vi "Image DAQ.vi"() -> ()   [LabVIEW 2020]
uses:
  SubVIs/MASTER.ctl
  SubVIs/Constants.ctl
  SubVIs/QBundle.ctl
  SubVIs/Queue.ctl
  SubVIs/Image data.ctl
  <vilib>/userdefined/High Color/IMAQdx.ctl
  <vilib>/vision/Image Controls.llb/IMAQ Image.ctl
  SubVIs/Image QBundle.ctl
panel:
  in  "Crosshairs":bool
  in  "Color Palette":u16(ring) items=["Grayscale U8", "False Color", "Overexposed"]
  in  "Exposure time [us]":dbl format="%#_10g"
  out "C2 Image out":T1(plugin-control) caption="Image Out"
  out "C2 Model Name":string
  in  "Camera 2":refnum<k21> caption="IMAQdx Session"
  out "C1 Image out":T1(plugin-control) caption="Image Out"
  out "C1 Model Name":string
  in  "Camera 1":refnum<k21> caption="IMAQdx Session"
  out "Image count":dbl
  in  "Digital output task":refnum<k21>
  in  "File type":string(combo)
  in  "Analog input task":refnum<k21>
  in  "Chart display tabs":T2(tab) caption="Display tabs"
  out "Analog Signals - Raw voltage":cluster{"Raw data[0]":dbl, "Raw data[1]":dbl}(graph)
  out "Analog Signals - Engineering units":cluster{"Engr data[0]":dbl, "Engr data[1]":dbl}(graph)
  in  "Scale (0) & Offset (1)":dbl[][](array[numeric])
  in  "AS #":string[](array[string])
  out "Channel Name":string[](array[string])
  out "Zero [V]":dbl[](array[numeric])
  out "Scale (0) & Offset (1)":dbl[][](array[numeric])
  in  "Enable":bool
  in  "Zero button":bool
  in  "Zero Signal [V]":dbl[](array[numeric])
  out "Analog Signals - Zero voltage":cluster{"Raw data[0]":dbl, "Raw data[1]":dbl}(graph)
  in  "Time":u16(ring) items=["Absolute time", "Relative time"]
  out "Timestamp [s]":dbl
  in  "Record data":bool
  in  "Sampling frequency [Hz]":dbl format="%#_10g"
  in  "Stop":bool
  in  "File Folder":path
  # "Records analog data and triggers cameras at specified rate. Writes raw voltage data to CSV file. Exports images as PNG files."
  # "Recording parameters- do not change while program is running"
  # "Recording indicators"
  # "Recording controls"
  # "Camera controls"
  # "Instructions: \n1. Click file icon to select file folder\n2. Select file type. Default is a CSV file. \n3. Set the sample frequency for data acquisition. Default is 1 Hz. \n4. Select analog input task\n5. Select digital output task\n6. Select type of timestamp\n7. Run program with white arrow in tool bar\n8. Use controls to record data adn trigger cameras\n9. Zero raw data on 'ZERO' tab. Zeroed data is recorded as raw data when 'Enable' button is on. \n10. Scale chart to engineering units on 'ENGR' tab\n11. Record AS number of equipment on 'Channel Info' tab\n12. Stop program with 'STOP' button"
  # "Note: If editing number of channels in DAQmx task, seek help from Instrumentation team. Chart cluster size & historical data constant must be adjusted in back panel."
  # "Scale [Unit/V] & Offset [Unit]"
  # "Channel Information"
  # "Offset [Unit]"
  # "Scale [Unit/V]"
  # "Zeroed data is recorded as raw data when Enable button is on."
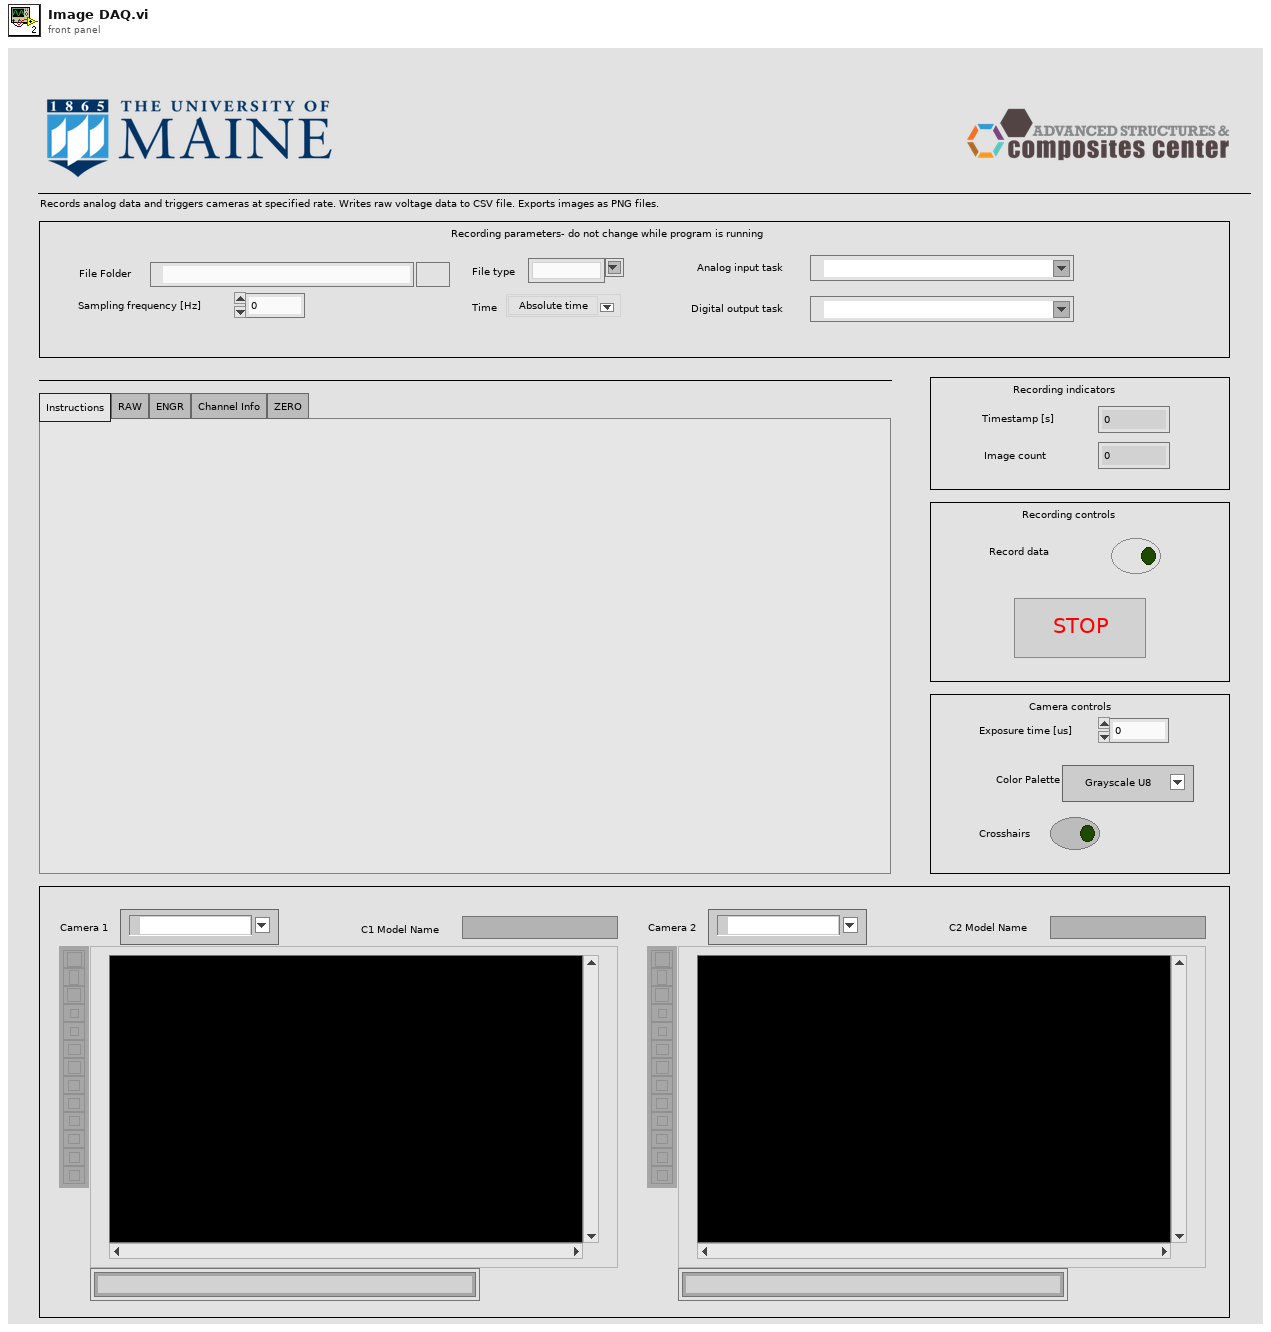
[diagram p1: front panel]
types:
  T1 = typedef "IMAQ Image.ctl" = refnum<image>
  T2 = enum32{"Instructions", "RAW", "ENGR", "Channel Info", "ZERO"}
  T3 = typedef "MASTER.ctl" = cluster{"Constants":T4, "Queue Bundle":T5, "Queue":T6, "Image data":T7, "Image QBundle ":T9}
  T4 = typedef "Constants.ctl" = cluster{"Time":u16, "Samp. freq. [Hz]":dbl, "Samp. per chan.":i32, "Avg. div.":i32, "File path":path, "AI":refnum<k21>, "Loop 1 [Hz]":dbl, "Loop 2 [Hz]":dbl, "Loop 3 [Hz]":dbl, "Loop 1 [ms]":dbl, "Loop 2 [ms]":dbl, "Loop 3 [ms]":dbl, "Q1 buffer size":i32, "Q2 buffer size":i32, "File type":string, "Loop 4 [Hz]":dbl, "Loop 4 [ms]":dbl, "Channel Name":string[], "AS #":string[], "DO":refnum<k21>}
  T5 = typedef "QBundle.ctl" = cluster{"queue 1":refnum<queue>, "error 1":errorcluster, "queue 2":refnum<queue>, "error 2":errorcluster}
  T6 = typedef "Queue.ctl" = cluster{"Enable zero":bool, "Engr data [Unit]":dbl[], "Zero button":bool, "Zero [V]":dbl[], "Timestamp [s]":dbl, "Write sample":bool, "Record control":bool, "Stop":bool, "error":errorcluster, "Raw data [V]\n(all samples)":dbl[][], "Raw data [V]":dbl[], "Loop count":i64, "Initial time [s]":dbl, "Scale (0) & Offset (1)":dbl[][], "Image count":dbl}
  T7 = typedef "Image data.ctl" = cluster{"Camera 1":T8, "Camera 2":T8, "C1 Image out ":T1, "C2 Image out":T1, "C1 Model Name":string, "C2 Model Name":string, "Exposure time [us]":dbl, "Color Palette":u16, "C1 Buffer array":T1[], "Ready":bool, "C2 Buffer array":T1[], "Crosshairs":bool, "Stop":bool}
  T8 = typedef "IMAQdx.ctl" = refnum<k21>
  T9 = typedef "Image QBundle.ctl" = cluster{"queue 1":refnum<queue>, "error 1":errorcluster, "queue 2":refnum<queue>, "error 2":errorcluster}
  T10 = cluster{"Engr data[0]":dbl, "Engr data[1]":dbl}[]
  T11 = cluster{"Engr data [Unit][0]":dbl, "Engr data [Unit][1]":dbl}
  T12 = cluster{"Raw data [V][0]":dbl, "Raw data [V][1]":dbl}
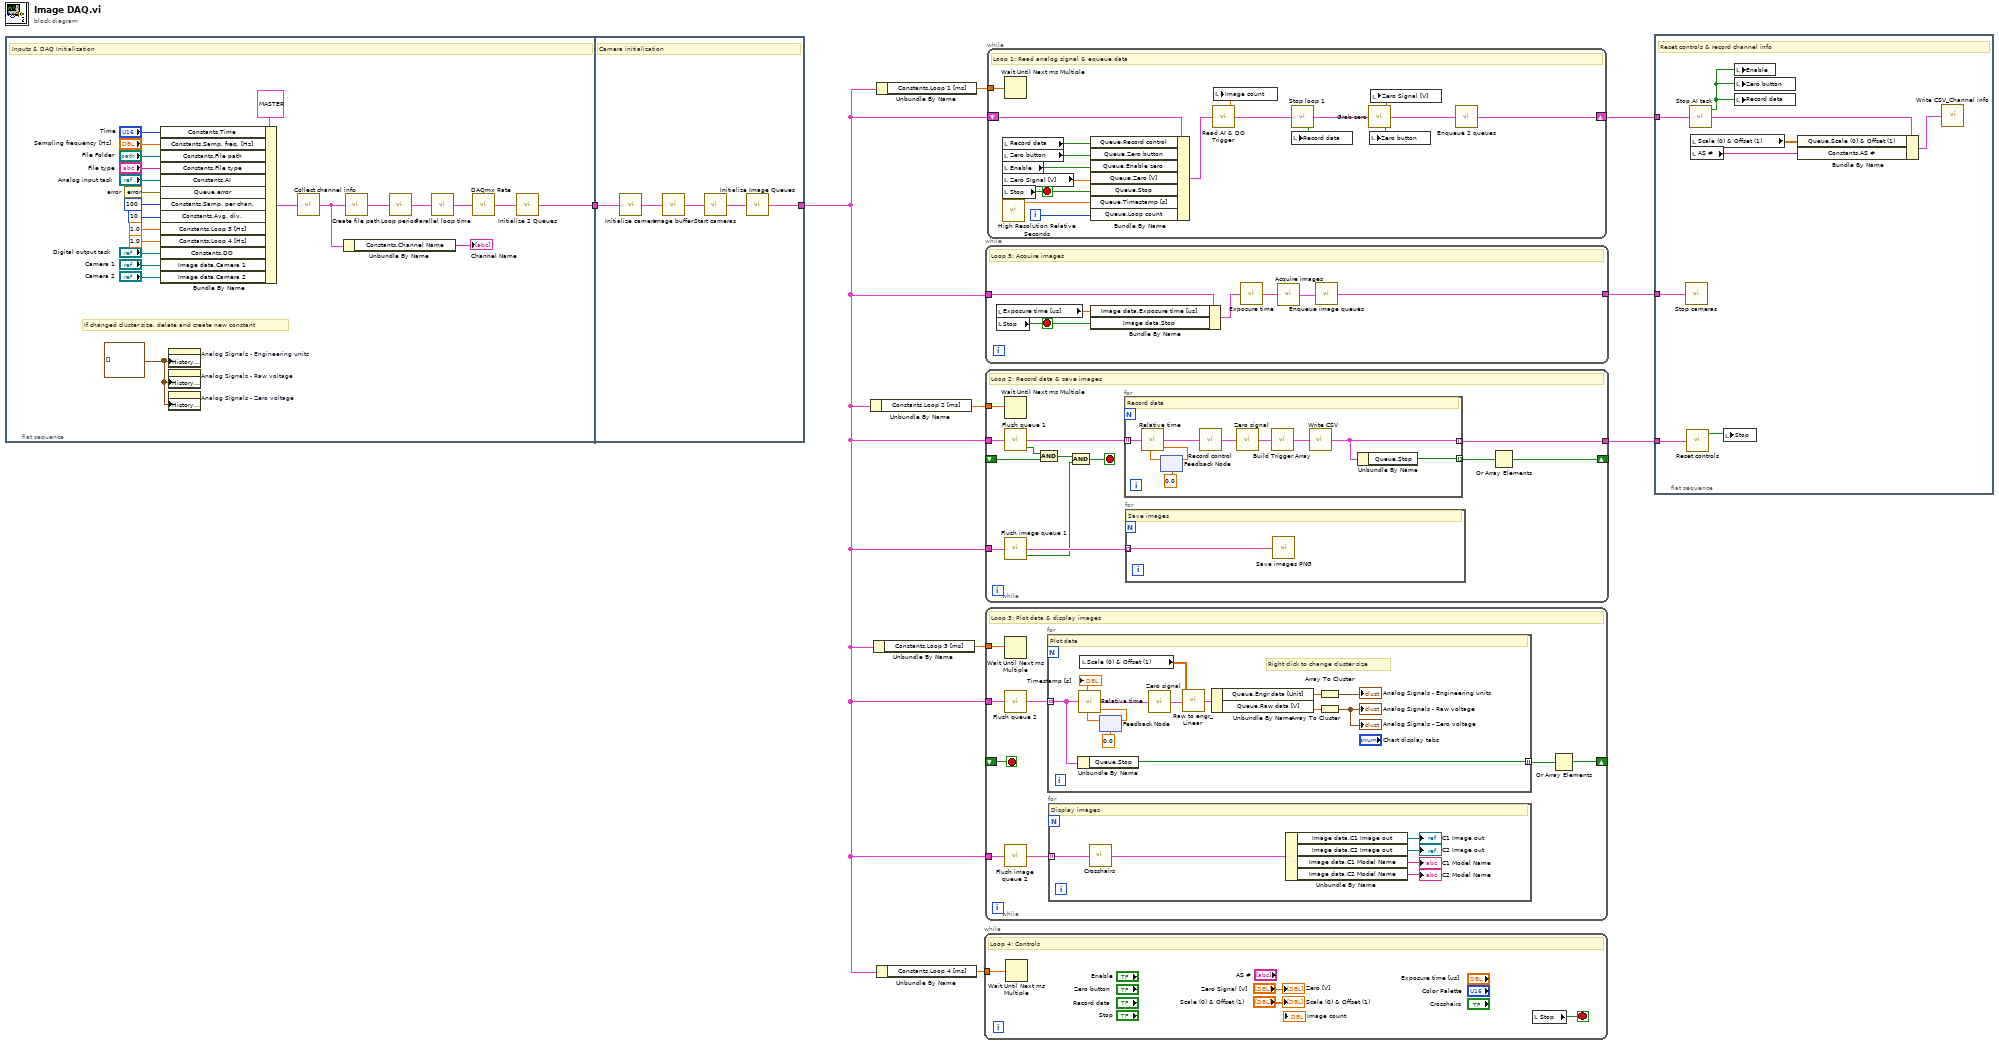
[diagram p0: block diagram]
diagram:
  n1 = flat-sequence {
    tunnel: [w32] -> w3
    tunnel: [w37] -> w1
    tunnel: w3 -> [w36]
    frame #0 {
      w20 = errorcluster {"status"=FALSE, "code"=0, "source"=""}  # error
      w31 = T10 [] ("History Data")
      # "If changed cluster size, delete and create new constant"
      # "Inputs & DAQ Initialization"
      n2 = Bundle By Name(cluster=T3 {"Constants"={"Time"=0, "Samp. freq. [Hz]"=0.0, "Samp. per chan."=0, "Avg. div."=0, "File path"=path "", "AI"="", "Loop 1 [Hz]"=0.0, "Loop 2 [Hz]"=0.0, "Loop 3 [Hz]"=0.0, "Loop 1 [ms]"=0.0, "Loop 2 [ms]"=0.0, "Loop 3 [ms]"=0.0, "Q1 buffer size"=0, "Q2 buffer size"=0, "File type"="", "Loop 4 [Hz]"=0.0, "Loop 4 [ms]"=0.0, "Channel Name"=[], "AS #"=[], "DO"=""}, "Queue Bundle"={"queue 1"=refnum, "error 1"={"status"=FALSE, "code"=0, "source"=""}, "queue 2"=refnum, "error 2"={"status"=FALSE, "code"=0, "source"=""}}, "Queue"={"Enable zero"=FALSE, "Engr data [Unit]"=[], "Zero button"=FALSE, "Zero [V]"=[], "Timestamp [s]"=0.0, "Write sample"=FALSE, "Record control"=FALSE, "Stop"=FALSE, "error"={"status"=FALSE, "code"=0, "source"=""}, "Raw data [V]\n(all samples)"=[], "Raw data [V]"=[], "Loop count"=0, "Initial time [s]"=0.0, "Scale (0) & Offset (1)"=[], "Image count"=0.0}, "Image data"={"Camera 1"="", "Camera 2"="", "C1 Image out "=refnum, "C2 Image out"=refnum, "C1 Model Name"="", "C2 Model Name"="", "Exposure time [us]"=0.0, "Color Palette"=0, "C1 Buffer array"=[], "Ready"=FALSE, "C2 Buffer array"=[], "Crosshairs"=FALSE, "Stop"=FALSE}, "Image QBundle "={"queue 1"=refnum, "error 1"={"status"=FALSE, "code"=0, "source"=""}, "queue 2"=refnum, "error 2"={"status"=FALSE, "code"=0, "source"=""}}} ("Variables"), "Constants.Time"="Time", "Constants.Samp. freq. [Hz]"="Sampling frequency [Hz]", "Constants.File path"="File Folder", "Constants.File type"="File type", "Constants.AI"="Analog input task", "Queue.error"=w20, "Constants.Samp. per chan."=100 ("Samp. per chan."), "Constants.Avg. div."=10 ("Avg. div."), "Constants.Loop 3 [Hz]"=1.0 ("Loop 1 [ms]"), "Constants.Loop 4 [Hz]"=1.0 ("Loop 4 [Hz]"), "Constants.DO"="Digital output task", "Image data.Camera 1"="Camera 1", "Image data.Camera 2"="Camera 2") -> (w15:T3)
      n3 = property on="Analog Signals - Engineering units" class="WFChart (strict)"("History Data"=w31) -> ()  [unwired: 2 in, 2 out]
      n4 = property on="Analog Signals - Raw voltage" class="WFChart (strict)"("History Data"=w31) -> ()  [unwired: 2 in, 2 out]
      n5 = property on="Analog Signals - Zero voltage" class="WFChart (strict)"("History Data"=w31) -> ()  [unwired: 2 in, 2 out]
      n6 = call "Collect channel info.vi"("MASTER in"=w15) -> ("MASTER out"=w13:T3)  [unwired: 4 in]
      n7 = Unbundle By Name(w13) -> ("Constants.Channel Name"=→"Channel Name":string[])
      n8 = call "Create file path.vi"("MASTER in"=w13) -> ("MASTER out"=w29:T3)  [unwired: 4 in]
      n9 = call "Loop period.vi"("MASTER in"=w29) -> ("MASTER out"=w26:T3)  [unwired: 4 in]
      n10 = call "Parallel loop time.vi"("MASTER in"=w26) -> ("MASTER out"=w30:T3)  [unwired: 4 in]
      n11 = call "DAQmx Rate.vi"("MASTER in"=w30) -> ("MASTER out"=w14:T3)  [unwired: 4 in]
      n12 = call "Initialize 2 Queues.vi"("MASTER in"=w14) -> ("MASTER out"=w32:T3)  [unwired: 4 in]
    }
    frame #1 {
      # "Camera initialization"
      n13 = call "Initialize camera.vi"("MASTER in"=w36) -> ("MASTER out"=w35:T3)  [unwired: 4 in]
      n14 = call "Image buffer.vi"("MASTER in"=w35) -> ("MASTER out"=w34:T3)  [unwired: 4 in]
      n15 = call "Start cameras.vi"("MASTER in"=w34) -> ("MASTER out"=w33:T3)  [unwired: 4 in]
      n16 = call "Initialize Image Queues.vi"("MASTER in"=w33) -> ("MASTER out"=w37:T3)  [unwired: 4 in]
    }
  }
  n17 = Unbundle By Name(w1) -> ("Constants.Loop 2 [ms]"=w6:dbl)
  n18 = Unbundle By Name(w1) -> ("Constants.Loop 3 [ms]"=w5:dbl)
  n19 = Unbundle By Name(w1) -> ("Constants.Loop 1 [ms]"=w7:dbl)
  n20 = Unbundle By Name(w1) -> ("Constants.Loop 4 [ms]"=w4:dbl)
  n21 = while {
    tunnel: w4 -> [w41]
    stop <- w38 stop-if-true
    # "Loop 4: Controls"
    n22 = Wait Until Next ms Multiple(millisecond multiple=w41) -> ()  [unwired: 1 out]
    n23 = local read "Stop"() -> (w38:bool)
    "Scale (0) & Offset (1)" <- "Scale (0) & Offset (1)"
    "Zero [V]" <- "Zero Signal [V]"
  }
  n24 = while {
    tunnel: w1 -> [w48]
    tunnel: [w42] -> w2
    stop <- w45 stop-if-true
    # "Loop 5: Acquire images"
    n25 = local read "Exposure time [us]"() -> (w46:dbl)
    n26 = local read "Stop"() -> (w45:bool)
    n27 = Bundle By Name(cluster=w48, "Image data.Exposure time [us]"=w46, "Image data.Stop"=w45) -> (w47:T3)
    n28 = call "Exposure time.vi"("MASTER in"=w47) -> ("MASTER out"=w44:T3)  [unwired: 4 in]
    n29 = call "Acquire images.vi"("MASTER in"=w44) -> ("MASTER out"=w43:T3)  [unwired: 4 in]
    n30 = call "Enqueue image queues.vi"("MASTER in"=w43) -> ("MASTER out"=w42:T3)  [unwired: 4 in]
  }
  n31 = while {
    tunnel: w6 -> [w61]
    shift-right: [w59] -> _
    shift-left: _ -> [w58]
    tunnel: w1 -> [w57]
    tunnel: [w54] -> w8
    tunnel: w1 -> [w52]
    stop <- w51 stop-if-true
    # "Loop 2: Record data & save images"
    n32 = Wait Until Next ms Multiple(millisecond multiple=w61) -> ()  [unwired: 1 out]
    n33 = call "Flush queue 1.vi"("MASTER in"=w57) -> ("MASTER array"=w55:T3[], "Zero elements in queue"=w56:bool)  [unwired: 5 in]
    n34 = call "Flush image queue 1.vi"("MASTER in"=w52) -> ("Zero elements in queue"=w49:bool, "MASTER array"=w53:T3[])  [unwired: 3 in]
    n35 = And(x=w56, y=w58) -> (x .and. y?=w50:bool)
    n36 = And(x=w50, y=w49) -> (x .and. y?=w51:bool)
    n37 = for {
      tunnel: [w72] -> w60 mode=indexing
      tunnel: w55 -> [w69] mode=indexing
      tunnel: [w70] -> w54 mode=indexing
      # "Record data"
      n38 = feedback #1(0.0 ("Initial time out")) -> (w65:dbl)
      n39 = call "Relative time.vi"("MASTER in"=w69, "Initial time in"=w65) -> ("Initial time out"=w66:dbl, "MASTER out"=w68:T3)  [unwired: 3 in, 1 out]
      n40 = feedback-in #1(w66) -> ()
      n41 = call "Record control.vi"("MASTER in"=w68) -> ("MASTER out"=w71:T3)  [unwired: 4 in]
      n42 = call "Zero signal.vi"("MASTER in"=w71) -> ("MASTER out"=w64:T3)  [unwired: 6 in]
      n43 = call "Build Trigger Array.vi"("MASTER in"=w64) -> ("MASTER out"=w63:T3)  [unwired: 4 in]
      n44 = call "Write CSV.vi"("MASTER in"=w63) -> ("MASTER out"=w70:T3)  [unwired: 4 in]
      n45 = Unbundle By Name(w70) -> ("Queue.Stop"=w72:bool)
    }
    n46 = for {
      tunnel: w53 -> [w62] mode=indexing
      # "Save images"
      n47 = call "Save images PNG.vi"("MASTER in"=w62) -> ()  [unwired: 4 in, 1 out]
    }
    n48 = Or Array Elements(Boolean array=w60) -> (logical OR=w59:bool)
  }
  n49 = while {
    tunnel: w5 -> [w80]
    shift-right: [w78] -> _
    shift-left: _ -> [w77]
    tunnel: w1 -> [w75]
    tunnel: w1 -> [w74]
    stop <- w77 stop-if-true
    # "Loop 3: Plot data & display images"
    n50 = Wait Until Next ms Multiple(millisecond multiple=w80) -> ()  [unwired: 1 out]
    n51 = call "Flush queue 2.vi"("MASTER in"=w75) -> ("MASTER array"=w76:T3[])  [unwired: 3 in, 1 out]
    n52 = call "Flush image queue 2.vi"("MASTER in"=w74) -> ("MASTER array"=w73:T3[])  [unwired: 3 in, 1 out]
    n53 = for {
      tunnel: w76 -> [w97] mode=indexing
      tunnel: [w100] -> w79 mode=indexing
      # "Right click to change cluster size"
      # "Plot data"
      n54 = Unbundle By Name(w97) -> ("Queue.Stop"=w100:bool)
      n55 = local read "Scale (0) & Offset (1)"() -> (w91:dbl[][])
      n56 = feedback #2(0.0 ("Initial time out")) -> (w94:dbl)
      n57 = call "Relative time.vi"("MASTER in"=w97, "Initial time in"=w94) -> ("Timestamp"=→"Timestamp [s]":dbl, "Initial time out"=w96:dbl, "MASTER out"=w93:T3)  [unwired: 3 in]
      n58 = feedback-in #2(w96) -> ()
      n59 = call "Zero signal.vi"("MASTER in"=w93) -> ("MASTER out"=w92:T3)  [unwired: 6 in]
      n60 = call "Raw to engr_Linear.vi"("MASTER in"=w92, "Slope (0) & Offset (1)"=w91) -> ("MASTER out"=w90:T3)  [unwired: 3 in]
      n61 = Unbundle By Name(w90) -> ("Queue.Engr data [Unit]"=w88:dbl[], "Queue.Raw data [V]"=w89:dbl[])
      n62 = Array To Cluster(array=w88) -> (cluster=→"Analog Signals - Engineering units":T11)
      n63 = Array To Cluster(array=w89) -> (cluster=→"Analog Signals - Raw voltage" →"Analog Signals - Zero voltage":T12)
    }
    n64 = for {
      tunnel: w73 -> [w82] mode=indexing
      # "Display images"
      n65 = call "Crosshairs.vi"("MASTER in"=w82) -> ("MASTER out"=w81:T3)  [unwired: 4 in]
      n66 = Unbundle By Name(w81) -> ("Image data.C1 Image out"=→"C1 Image out":T1, "Image data.C2 Image out"=→"C2 Image out":T1, "Image data.C1 Model Name"=→"C1 Model Name":string, "Image data.C2 Model Name"=→"C2 Model Name":string)
    }
    n67 = Or Array Elements(Boolean array=w79) -> (logical OR=w78:bool)
  }
  n68 = while {
    tunnel: w7 -> [w118]
    shift-right: [w107] -> w9
    shift-left: w1 -> [w104]
    i -> [w109]
    stop <- w110 stop-if-true
    # "Loop 1: Read analog signal & equeue data"
    n69 = local read "Record data"() -> (w112:bool)
    n70 = local read "Zero button"() -> (w115:bool)
    n71 = local read "Enable"() -> (w114:bool)
    n72 = local read "Zero Signal [V]"() -> (w113:dbl[])
    n73 = local read "Stop"() -> (w110:bool)
    n74 = call <vilib>:"High Resolution Relative Seconds.vi"() -> ("relative seconds"=w117:dbl)
    n75 = Wait Until Next ms Multiple(millisecond multiple=w118) -> ()  [unwired: 1 out]
    n76 = Bundle By Name(cluster=w104, "Queue.Record control"=w112, "Queue.Zero button"=w115, "Queue.Enable zero"=w114, "Queue.Zero [V]"=w113, "Queue.Stop"=w110, "Queue.Timestamp [s]"=w117, "Queue.Loop count"=w109) -> (w103:T3)
    n77 = call "Read AI & DO Trigger.vi"("MASTER in"=w103) -> ("MASTER out"=w102:T3, "Image count"=w101:dbl)  [unwired: 3 in]
    n78 = local write "Image count"(w101) -> ()
    n79 = call "Stop loop 1.vi"("MASTER in"=w102) -> ("Record out"=w106:bool, "MASTER out"=w105:T3)  [unwired: 3 in]
    n80 = local write "Record data"(w106) -> ()
    n81 = call "Grab zero.vi"("MASTER in"=w105) -> ("Zero button"=w111:bool, "MASTER out"=w108:T3, "Zeros"=w116:dbl[])  [unwired: 2 in]
    n82 = local write "Zero button"(w111) -> ()
    n83 = local write "Zero Signal [V]"(w116) -> ()
    n84 = call "Enqueue 2 queues.vi"("MASTER in"=w108) -> ("MASTER out"=w107:T3)  [unwired: 4 in]
  }
  n85 = flat-sequence {
    tunnel: w9 -> [w127]
    tunnel: w8 -> [w121]
    tunnel: w2 -> [w119]
    frame #0 {
      # "Reset controls & record channel info"
      n86 = call "Stop cameras.vi"("MASTER in"=w119) -> ()  [unwired: 5 in]
      n87 = call "Reset controls.vi"("MASTER Array in"=w121) -> ("Reset controls (F)"=w120:bool)  [unwired: 3 in, 1 out]
      n88 = call "Stop AI task.vi"("MASTER in"=w127) -> ("MASTER out"=w124:T3, "Reset controls (F)"=w126:bool)  [unwired: 3 in]
      n89 = local read "Scale (0) & Offset (1)"() -> (w125:dbl[][])
      n90 = local read "AS #"() -> (w123:string[])
      n91 = local write "Stop"(w120) -> ()
      n92 = local write "Enable"(w126) -> ()
      n93 = local write "Zero button"(w126) -> ()
      n94 = local write "Record data"(w126) -> ()
      n95 = Bundle By Name(cluster=w124, "Queue.Scale (0) & Offset (1)"=w125, "Constants.AS #"=w123) -> (w122:T3)
      n96 = call "Write CSV_Channel info.vi"("MASTER in"=w122) -> ()  [unwired: 4 in, 1 out]
    }
  }
